vi "Linked Network Actor Test.vi"() -> ()   [LabVIEW 2014]
uses:
  <vilib>/NI/Actors/Linked Network Actor/Linked Network Actor/Linked Network Actor.lvclass
  <vilib>/ActorFramework/Message Enqueuer/Message Enqueuer.lvclass
  <vilib>/ActorFramework/Message Queue/Message Queue.lvclass/Message Queue.ctl
  <vilib>/ActorFramework/Message Dequeuer/Message Dequeuer.lvclass/Message Dequeuer.ctl
  Loopback/Loopback.lvclass
  <vilib>/NI/Actors/Linked Network Actor/Linked Network Actor Messages/LNA Connection Status Msg/LNA Connection Status Msg.lvclass
  <vilib>/NI/Actors/Linked Network Actor/Linked Network Actor Messages/LNA Connection Status Msg/LNA Connection Status Msg.lvclass/LNA Connection Status Msg.ctl
  <vilib>/NI/Actors/Linked Network Actor/Linked Network Actor Messages/LNA Return Message Msg/LNA Return Message Msg.lvclass
  <vilib>/ActorFramework/LastAck/Last Ack.lvclass
  <vilib>/ActorFramework/LastAck/Last Ack.lvclass/Last Ack.ctl
  <vilib>/ActorFramework/Message Enqueuer/Message Enqueuer.lvclass/Message Enqueuer.ctl
  <vilib>/ActorFramework/Message Enqueuer/Enqueue.vi
  <vilib>/ActorFramework/Message Priority Queue/Priority Dequeue.vi
  <vilib>/ActorFramework/Message Priority Queue/Priority Enqueue.vi
  <vilib>/ActorFramework/Stop Msg/Stop Msg.lvclass
  <vilib>/ActorFramework/Message/Message.lvclass
  <vilib>/ActorFramework/Actor/Actor.lvclass
  <vilib>/ActorFramework/Message Queue/Message Queue.lvclass
  <vilib>/ActorFramework/Message Dequeuer/Message Dequeuer.lvclass
  <vilib>/NI/Actors/Linked Network Actor/Linked Network Actor Messages/Disconnect Msg/Disconnect Msg.lvclass
  <vilib>/NI/Actors/Linked Network Actor/Linked Network Actor Messages/Connect Msg/Connect Msg.lvclass
  <vilib>/NI/Actors/Linked Network Actor/Linked Network Actor Messages/Transmit Network Message Msg/Transmit Network Message Msg.lvclass
panel:
  out "Returned Err":errorcluster
  out "Returned Paths":path[](array[path])
  out "Returned Times":timestamp[](array[timestamp])
  in  "Open Actor Core front panels? (F)":bool
  in  "Start B":bool
  in  "Start A":bool
  out "name":string
  out "Disconnected":string
  in  "Stop B":bool
  in  "Stop A":bool
  in  "stop":bool
  out "Writer B":bool
  out "Reader B":bool
  out "Reader A":bool
  out "Writer A":bool
  in  "Disconnect B":bool
  in  "Connect B":bool
  in  "Disconnect A":bool
  in  "Connect A":bool
  out "Paths":path[](array[path])
  out "Times":timestamp[](array[timestamp]) format="%<%.3X>T"
  in  "Send B":bool
  in  "Send A":bool
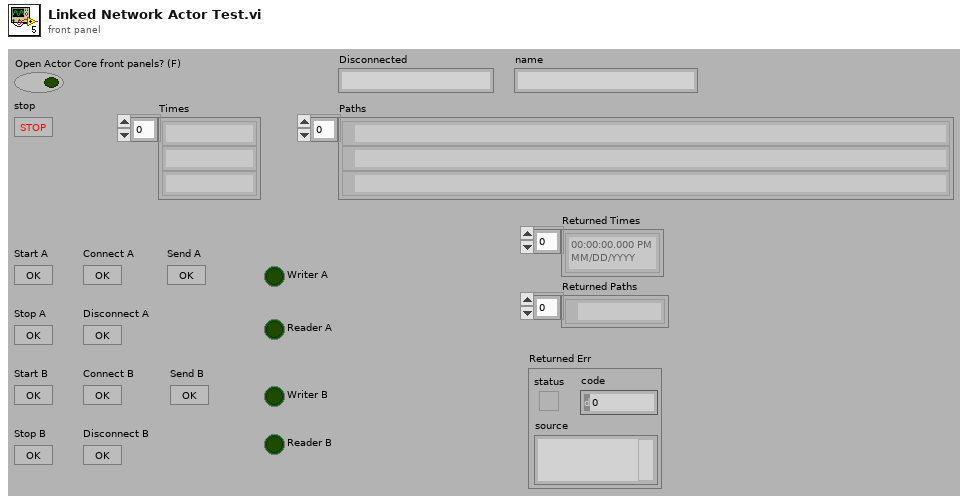
[diagram p1: front panel]
types:
  T1 = typedef "Actor Framework.lvlib/Message Enqueuer.lvclass/Message Priority.ctl" = enum16{"Low", "Normal", "High"}
  T2 = cluster{"Tx Message":refnum<class "Message.lvclass">, "Tx Error":errorcluster, "Message Priority":T1}
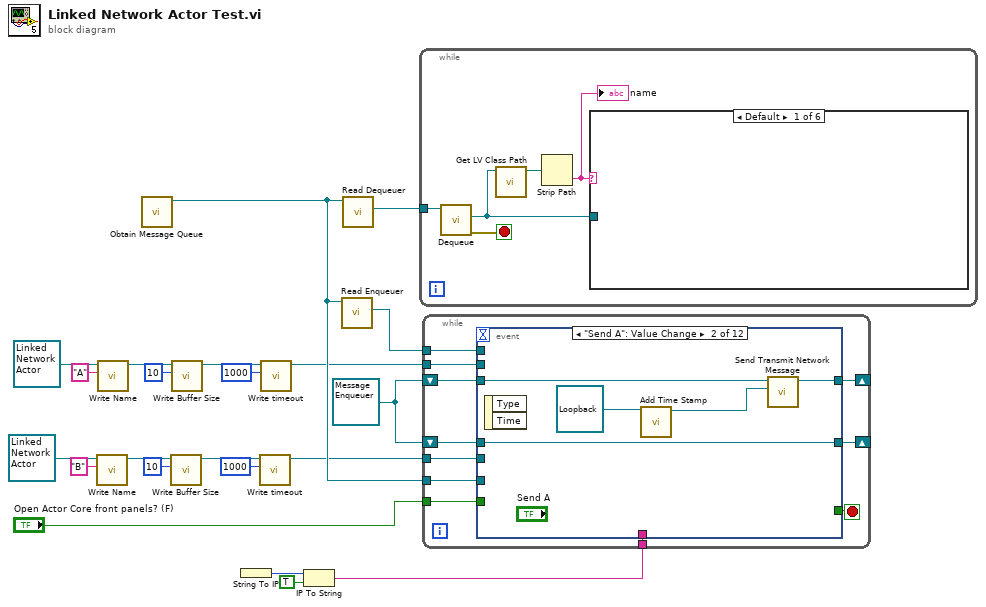
[diagram p0: block diagram]
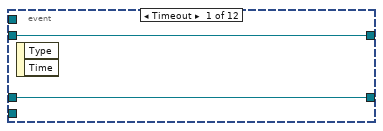
[diagram p2: hidden frame]
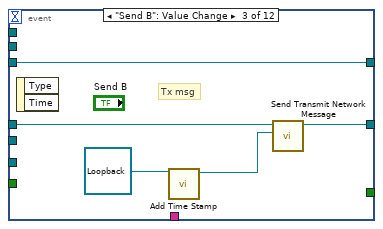
[diagram p3: hidden frame]
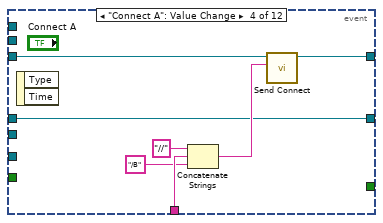
[diagram p4: hidden frame]
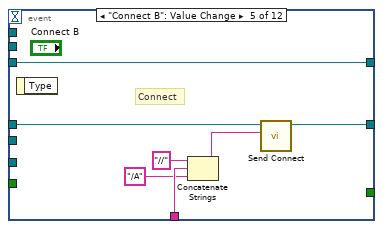
[diagram p5: hidden frame]
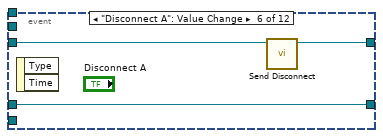
[diagram p6: hidden frame]
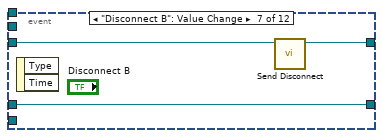
[diagram p7: hidden frame]
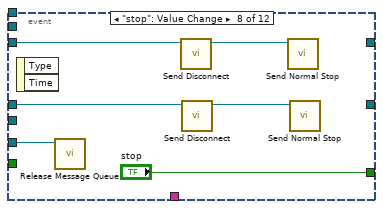
[diagram p8: hidden frame]
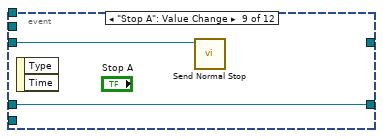
[diagram p9: hidden frame]
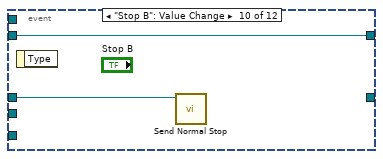
[diagram p10: hidden frame]
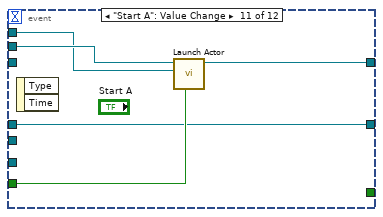
[diagram p11: hidden frame]
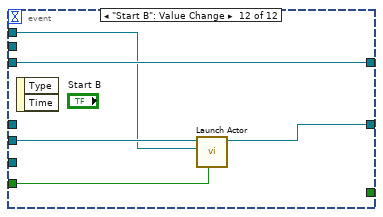
[diagram p12: hidden frame]
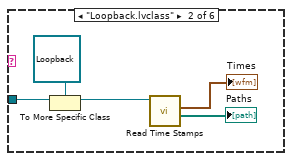
[diagram p13: hidden frame]
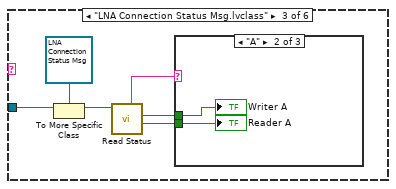
[diagram p14: hidden frame]
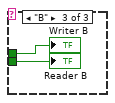
[diagram p16: hidden frame]
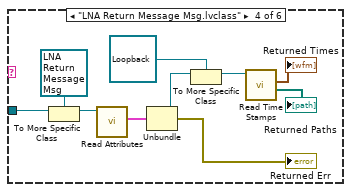
[diagram p17: hidden frame]
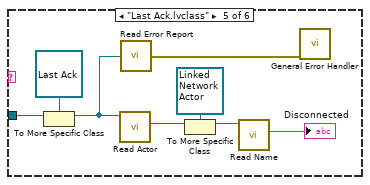
[diagram p18: hidden frame]
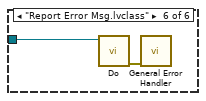
[diagram p19: hidden frame]
diagram:
  w1 = refnum<class "Message Enqueuer.lvclass"> refnum ("Caller-To-Actor Enqueuer")
  n1 = call <vilib>:"Write Name.vi"("Name"="B", "Network Actor in"=refnum<class "Linked Network Actor.lvclass"> refnum ("Network Actor.lvlib:Network Actor.lvclass")) -> ("Network Actor out"=w15:refnum<class "Linked Network Actor.lvclass">)  [unwired: 9 in]
  n2 = call <vilib>:"Write Name.vi"("Name"="A", "Network Actor in"=refnum<class "Linked Network Actor.lvclass"> refnum ("Network Actor.lvlib:Network Actor.lvclass")) -> ("Network Actor out"=w21:refnum<class "Linked Network Actor.lvclass">)  [unwired: 9 in]
  n3 = call <vilib>:"Obtain Message Queue.vi"() -> ("Message Queue"=w6:refnum<class "Message Queue.lvclass">)  [unwired: 10 in, 1 out]
  n4 = call <vilib>:"Write Buffer Size.vi"("Buffer Size"=10, "Network Actor in"=w15) -> ("Network Actor out"=w14:refnum<class "Linked Network Actor.lvclass">)  [unwired: 9 in]
  n5 = call <vilib>:"Write Buffer Size.vi"("Buffer Size"=10, "Network Actor in"=w21) -> ("Network Actor out"=w20:refnum<class "Linked Network Actor.lvclass">)  [unwired: 9 in]
  n6 = String To IP() -> (0:w9:u32)  [unwired: 1 in]
  n7 = call <vilib>:"Write timeout.vi"("timeout"=1000, "Network Actor in"=w14) -> ("Network Actor out"=w4:refnum<class "Linked Network Actor.lvclass">)  [unwired: 9 in]
  n8 = call <vilib>:"Write timeout.vi"("timeout"=1000, "Network Actor in"=w20) -> ("Network Actor out"=w5:refnum<class "Linked Network Actor.lvclass">)  [unwired: 9 in]
  n9 = IP To String(1:TRUE ("dot notation? (F)"), 2:w9) -> (0:w8:string)
  n10 = call <vilib>:"Read Enqueuer.vi"("Message Queue"=w6) -> ("Message Enqueuer"=w2:refnum<class "Message Enqueuer.lvclass">)  [unwired: 10 in]
  n11 = call <vilib>:"Read Dequeuer.vi"("Message Queue"=w6) -> ("Message Dequeuer"=w7:refnum<class "Message Dequeuer.lvclass">)  [unwired: 10 in]
  n12 = while {
    tunnel: w7 -> [w26]
    stop <- w24 stop-if-true
    n13 = call <vilib>:"Dequeue.vi"("Message Dequeuer in"=w26) -> ("error out"=w24:errorcluster, "Message"=w25:refnum<class "Message.lvclass">)  [unwired: 6 in, 3 out]
    n14 = call <vilib>:"Get LV Class Path.vi"("object"=w25) -> ("class path"=w27:path)  [unwired: 9 in, 1 out]
    n15 = Strip Path(path=w27) -> (name=w23:string)  [unwired: 1 out]
    "name" <- w23
    n16 = case shown="Default" w23 {
      tunnel: w25 -> [_ w29 w38 w43 w60 w62]
      frame Default {
      }
      frame "Loopback.lvclass" {
        n17 = To More Specific Class(target class=refnum<class "Loopback.lvclass"> refnum ("Loopback.lvclass"), reference=w29) -> (specific class reference=w28:refnum<class "Loopback.lvclass">)  [unwired: 1 in, 1 out]
        n18 = call "Read Time Stamps.vi"("Loopback in"=w28) -> ("Paths"=→"Paths":path[], "Times"=→"Times":timestamp[])  [unwired: 7 in, 2 out]
      }
      frame "LNA Connection Status Msg.lvclass" {
        n19 = To More Specific Class(target class=refnum<class "LNA Connection Status Msg.lvclass"> refnum ("Linked Network Actor.lvlib:LNA Connection Status Msg.lvclass"), reference=w38) -> (specific class reference=w37:refnum<class "LNA Connection Status Msg.lvclass">)  [unwired: 1 in, 1 out]
        n20 = call <vilib>:"Read Status.vi"("Update Status Msg in"=w37) -> ("Reader"=w34:bool, "Writer"=w35:bool, "Name"=w36:string)  [unwired: 7 in, 1 out]
        n21 = case shown="\"A\"" w36 {
          tunnel: w35 -> [_ w40 w42]
          tunnel: w34 -> [_ w39 w41]
          frame Default {
          }
          frame "A" {
            "Writer A" <- w40
            "Reader A" <- w39
          }
          frame "B" {
            "Writer B" <- w42
            "Reader B" <- w41
          }
        }
      }
      frame "LNA Return Message Msg.lvclass" {
        n22 = To More Specific Class(target class=refnum<class "LNA Return Message Msg.lvclass"> refnum ("Linked Network Actor.lvlib:LNA Return Message Msg.lvclass"), reference=w43) -> (specific class reference=w51:refnum<class "LNA Return Message Msg.lvclass">)  [unwired: 1 in, 1 out]
        n23 = call <vilib>:"Read Attributes.vi"("Abstract Message Template in"=w51) -> ("Payload"=w50:T2)  [unwired: 9 in, 1 out]
        n24 = Unbundle(w50) -> ("Tx Message"=w47:refnum<class "Message.lvclass">, "Tx Error"=→"Returned Err":errorcluster)  [unwired: 1 out]
        n25 = To More Specific Class(target class=refnum<class "Loopback.lvclass"> refnum ("Loopback.lvclass"), reference=w47) -> (specific class reference=w48:refnum<class "Loopback.lvclass">)  [unwired: 1 in, 1 out]
        n26 = call "Read Time Stamps.vi"("Loopback in"=w48) -> ("Paths"=→"Returned Paths":path[], "Times"=→"Returned Times":timestamp[])  [unwired: 7 in, 2 out]
      }
      frame "Last Ack.lvclass" {
        n27 = To More Specific Class(target class=refnum<class "Last Ack.lvclass"> refnum ("Actor Framework.lvlib:Last Ack.lvclass"), reference=w60) -> (specific class reference=w54:refnum<class "Last Ack.lvclass">)  [unwired: 1 in, 1 out]
        n28 = call <vilib>:"Read Actor.vi"("Last Ack"=w54) -> ("Actor"=w58:refnum<class "Actor.lvclass">)  [unwired: 10 in]
        n29 = call <vilib>:"Read Error Report.vi"("Last Ack"=w54) -> ("error report"=w53:errorcluster)
        n30 = To More Specific Class(target class=refnum<class "Linked Network Actor.lvclass"> refnum ("Network Actor.lvlib:Network Actor.lvclass"), reference=w58) -> (specific class reference=w56:refnum<class "Linked Network Actor.lvclass">)  [unwired: 1 in, 1 out]
        n31 = call-dynamic "Read Name.vi"("Network Actor in"=w56) -> ("Name"=→"Disconnected":string)  [unwired: 10 in]
        n32 = call <vilib>:"General Error Handler.vi"("error in (no error)"=w53) -> ()  [unwired: 10 in, 5 out]
      }
      frame "Report Error Msg.lvclass" {
        n33 = call-dynamic "Do.vi"("Message"=w62) -> ("error out"=w61:errorcluster)  [unwired: 9 in, 1 out]
        n34 = call <vilib>:"General Error Handler.vi"("error in (no error)"=w61) -> ()  [unwired: 10 in, 5 out]
      }
    }
  }
  n35 = while {
    tunnel: w8 -> [w71]
    tunnel: w6 -> [w69]
    shift-right: [w67] -> _
    shift-left: w1 -> [w73]
    tunnel: w5 -> [w68]
    shift-right: [w65] -> _
    shift-left: w1 -> [w72]
    tunnel: w4 -> [w66]
    tunnel: "Open Actor Core front panels? (F)" -> [w64]
    tunnel: w2 -> [w63]
    stop <- w70 stop-if-true
    n36 = event shown="[1] \"Send A\": Value Change" {
      selector: _ -> [_ _ _ _ _ _ _ _ _ _ _ _]
      dyn-events: _ -> [_ _ _ _ _ _ _ _ _ _ _ _]
      timeout: _ -> [_ _ _ _ _ _ _ _ _ _ _ _]
      tunnel: w73 -> [w74 w79 w82 w89 w94 w102 w105 w107 w113 w114 _ w122]
      tunnel: w72 -> [w75 w76 w84 w86 w95 w100 w103 w109 w112 w115 w116 _]
      tunnel: w71 -> [_ _ _ w92 w99 _ _ _ _ _ _ _]
      tunnel: [_ _ _ _ _ _ _ "stop" _ _ _ _] -> w70
      tunnel: w69 -> [_ _ _ _ _ _ _ w110 _ _ _ _]
      tunnel: w68 -> [_ _ _ _ _ _ _ _ _ _ w120 _]
      tunnel: [w74 w77 w82 w87 w94 w101 w104 _ _ w114 w119 w122] -> w67
      tunnel: w66 -> [_ _ _ _ _ _ _ _ _ _ _ w125]
      tunnel: [w75 w76 w81 w86 w93 w100 w103 _ w112 _ w116 w124] -> w65
      tunnel: w64 -> [_ _ _ _ _ _ _ _ _ _ w118 w123]
      tunnel: w63 -> [_ _ _ _ _ _ _ _ _ _ w117 w121]
      event Timeout {
        n37 = event-data() -> ()  [unwired: 1 in, 2 out]
      }
      event "Send A": Value Change {
        n38 = event-data() -> ()  [unwired: 1 in, 2 out]
        n39 = call "Add Time Stamp.vi"("Loopback in"=refnum<class "Loopback.lvclass"> refnum ("Loopback.lvclass")) -> ("Loopback out"=w78:refnum<class "Loopback.lvclass">)  [unwired: 9 in, 1 out]
        n40 = call <vilib>:"Send Transmit Network Message.vi"("Message"=w78, "Message Enqueuer"=w79) -> ("Message Enqueuer out"=w77:refnum<class "Message Enqueuer.lvclass">)  [unwired: 8 in, 1 out]
      }
      event "Send B": Value Change {
        # "Tx msg"
        n41 = event-data() -> ()  [unwired: 1 in, 2 out]
        n42 = call "Add Time Stamp.vi"("Loopback in"=refnum<class "Loopback.lvclass"> refnum ("Loopback.lvclass")) -> ("Loopback out"=w83:refnum<class "Loopback.lvclass">)  [unwired: 9 in, 1 out]
        n43 = call <vilib>:"Send Transmit Network Message.vi"("Message"=w83, "Message Enqueuer"=w84) -> ("Message Enqueuer out"=w81:refnum<class "Message Enqueuer.lvclass">)  [unwired: 8 in, 1 out]
      }
      event "Connect A": Value Change {
        n44 = event-data() -> ()  [unwired: 1 in, 2 out]
        n45 = Concatenate Strings("//" ("string"), w92, "/B" ("format string")) -> (w88:string)
        n46 = call <vilib>:"Send Connect.vi"("URL"=w88, "Message Enqueuer"=w89) -> ("Message Enqueuer out"=w87:refnum<class "Message Enqueuer.lvclass">)  [unwired: 8 in, 1 out]
      }
      event "Connect B": Value Change {
        # "Connect"
        n47 = event-data() -> ()  [unwired: 1 in, 1 out]
        n48 = Concatenate Strings("//" ("string"), w99, "/A" ("format string")) -> (w96:string)
        n49 = call <vilib>:"Send Connect.vi"("URL"=w96, "Message Enqueuer"=w95) -> ("Message Enqueuer out"=w93:refnum<class "Message Enqueuer.lvclass">)  [unwired: 8 in, 1 out]
      }
      event "Disconnect A": Value Change {
        n50 = event-data() -> ()  [unwired: 1 in, 2 out]
        n51 = call <vilib>:"Send Disconnect.vi"("Message Enqueuer"=w102) -> ("Message Enqueuer out"=w101:refnum<class "Message Enqueuer.lvclass">)  [unwired: 9 in, 1 out]
      }
      event "Disconnect B": Value Change {
        n52 = event-data() -> ()  [unwired: 1 in, 2 out]
        n53 = call <vilib>:"Send Disconnect.vi"("Message Enqueuer"=w105) -> ("Message Enqueuer out"=w104:refnum<class "Message Enqueuer.lvclass">)  [unwired: 9 in, 1 out]
      }
      event "stop": Value Change {
        n54 = event-data() -> ()  [unwired: 1 in, 2 out]
        n55 = call <vilib>:"Release Message Queue.vi"("Message Queue"=w110) -> ()  [unwired: 9 in, 2 out]
        n56 = call <vilib>:"Send Disconnect.vi"("Message Enqueuer"=w107) -> ("Message Enqueuer out"=w106:refnum<class "Message Enqueuer.lvclass">)  [unwired: 9 in, 1 out]
        n57 = call <vilib>:"Send Disconnect.vi"("Message Enqueuer"=w109) -> ("Message Enqueuer out"=w108:refnum<class "Message Enqueuer.lvclass">)  [unwired: 9 in, 1 out]
        n58 = call <vilib>:"Send Normal Stop.vi"("Message Enqueuer"=w106) -> ()  [unwired: 10 in, 1 out]
        n59 = call <vilib>:"Send Normal Stop.vi"("Message Enqueuer"=w108) -> ()  [unwired: 10 in, 1 out]
      }
      event "Stop A": Value Change {
        n60 = event-data() -> ()  [unwired: 1 in, 2 out]
        n61 = call <vilib>:"Send Normal Stop.vi"("Message Enqueuer"=w113) -> ()  [unwired: 10 in, 1 out]
      }
      event "Stop B": Value Change {
        n62 = event-data() -> ()  [unwired: 1 in, 1 out]
        n63 = call <vilib>:"Send Normal Stop.vi"("Message Enqueuer"=w115) -> ()  [unwired: 10 in, 1 out]
      }
      event "Start A": Value Change {
        n64 = event-data() -> ()  [unwired: 1 in, 2 out]
        n65 = call <vilib>:"Launch Actor.vi"("Open Actor Core front panel? (F)"=w118, "Actor-to-Caller Enqueuer"=w117, "Actor"=w120) -> ("Caller-To-Actor Enqueuer"=w119:refnum<class "Message Enqueuer.lvclass">)  [unwired: 7 in, 1 out]
      }
      event "Start B": Value Change {
        n66 = event-data() -> ()  [unwired: 1 in, 2 out]
        n67 = call <vilib>:"Launch Actor.vi"("Open Actor Core front panel? (F)"=w123, "Actor-to-Caller Enqueuer"=w121, "Actor"=w125) -> ("Caller-To-Actor Enqueuer"=w124:refnum<class "Message Enqueuer.lvclass">)  [unwired: 7 in, 1 out]
      }
    }
  }
